vi "MAIN_eq_2grado.vi"() -> ()   [LabVIEW 2021]
panel:
  out "XY Graph":cluster{"Y":dbl[], "Y":dbl[]}[](graph)
  out "Parte Immaginaria":cluster{"Im1":dbl, "Im2":dbl}
  out "Parte Reale":cluster{"Re1":dbl, "Re2":dbl}
  in  "Coefficienti":cluster{"a":i16, "b":i16, "c":i16}
  out "Tipo Radici":string
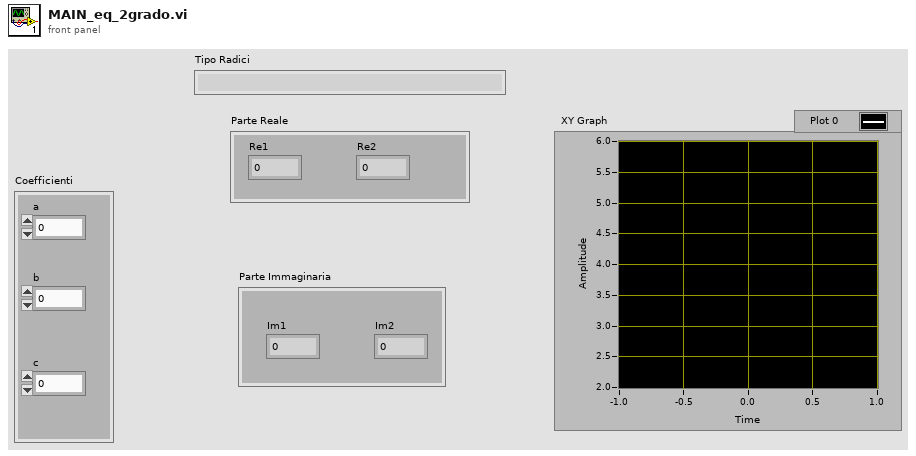
[diagram p1: front panel]
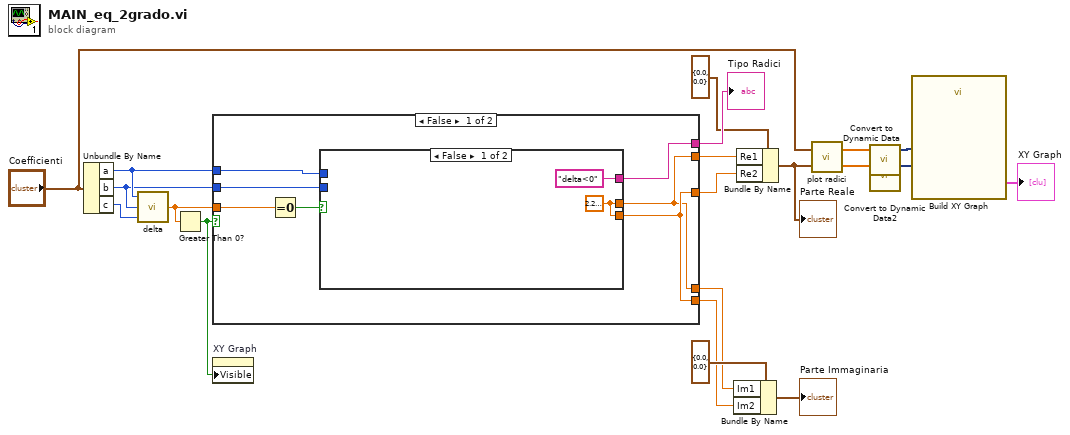
[diagram p0: block diagram]
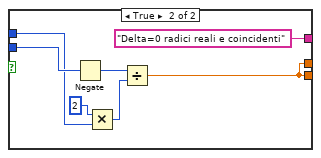
[diagram p2: hidden frame]
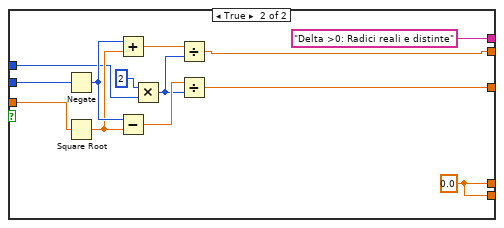
[diagram p3: hidden frame]
diagram:
  n1 = Unbundle By Name("Coefficienti") -> ("a"=w18:i16, "b"=w17:i16, "c"=w16:i16)
  n2 = call "delta.vi"("c"=w16, "b"=w17, "a"=w18) -> ("delta"=w19:dbl)
  n3 = Greater Than 0?(x=w19) -> (x > 0?=w1:bool)
  n4 = case shown="False" w1 {
    tunnel: [w23 "Delta >0: Radici reali e distinte"] -> w20
    tunnel: w17 -> [w25 w47]
    tunnel: w18 -> [w24 w44]
    tunnel: w19 -> [w27 w48]
    tunnel: [w21 w39] -> w10
    tunnel: [w22 w38] -> w9
    tunnel: [w22 w37] -> w13
    tunnel: [w21 w37] -> w12
    frame False {
      n5 = Equal To 0?(x=w27) -> (x = 0?=w26:bool)
      n6 = case shown="False" w26 {
        tunnel: w25 -> [_ w36]
        tunnel: w24 -> [_ w35]
        tunnel: ["delta<0" "Delta=0 radici reali e coincidenti"] -> w23
        tunnel: [w29 w30] -> w21
        tunnel: [w29 w30] -> w22
        frame False {
          w29 = 2.220446049250313e-16
        }
        frame True {
          n7 = Negate(x=w36) -> (-x=w33:i16)
          n8 = Multiply(x=2, y=w35) -> (x*y=w32:i32)
          n9 = Divide(x=w33, y=w32) -> (x/y=w30:dbl)
        }
      }
    }
    frame True {
      w37 = 0.0
      n10 = Negate(x=w47) -> (-x=w46:i16)
      n11 = Square Root(x=w48) -> (sqrt(x)=w45:dbl)
      n12 = Add(x=w46, y=w45) -> (x+y=w42:dbl)
      n13 = Subtract(x=w46, y=w45) -> (x-y=w41:dbl)
      n14 = Multiply(x=2, y=w44) -> (x*y=w40:i32)
      n15 = Divide(x=w42, y=w40) -> (x/y=w39:dbl)
      n16 = Divide(x=w41, y=w40) -> (x/y=w38:dbl)
    }
  }
  "Tipo Radici" <- w20
  n17 = property on="XY Graph" class="XYGraph (strict)"("Visible"=w1) -> ()  [unwired: 2 in, 2 out]
  n18 = Bundle By Name(cluster=cluster{"Im1":dbl, "Im2":dbl} {"Im1"=0.0, "Im2"=0.0} ("Parte Immaginaria 2"), "Im1"=w12, "Im2"=w13) -> (→"Parte Immaginaria":cluster{"Im1":dbl, "Im2":dbl})
  n19 = Bundle By Name(cluster=cluster{"Re1":dbl, "Re2":dbl} {"Re1"=0.0, "Re2"=0.0} ("Parte Reale"), "Re1"=w10, "Re2"=w9) -> (w7:cluster{"Re1":dbl, "Re2":dbl})
  "Parte Reale" <- w7
  n20 = call "plot radici.vi"("Parte Reale"=w7, "Coefficienti"="Coefficienti") -> ("Asse Y"=w3:dbl[], "Asse X"=w5:dbl[])
  n21 = call "Convert to Dynamic Data"("Array"=w5) -> ("Dynamic Data Type"=w4:dynamicdata)  [unwired: 3 in]
  n22 = call "Convert to Dynamic Data2"("Array"=w3) -> ("Dynamic Data Type"=w2:dynamicdata)  [unwired: 3 in]
  n23 = call "Build XY Graph"("Y Input"=w2, "X Input"=w4) -> ("XY Graph"=→"XY Graph":cluster{"X":dbl[], "Y":dbl[]}[])  [unwired: 8 in, 1 out]
